vi "SwapInstanceVIUnusedName2 61.vi"(6 "Bindata & descr in":T1, 7 "type":i16, 8 "error in (no error)":errorcluster, 9 "dims":u8=3 min=1 max=3, 11 "kwarg_name":string="testarg") -> (0 "error out":errorcluster, 1 "Array 3D":i16[][][](array[numeric]), 2 "Array 2D":i16[][](array[numeric]), 3 "Array 1D":i16[](array[numeric]), 4 "Bindata & descr out":T1, 5 "bindata":u8[](array[numeric]))   [LabVIEW 2018]
uses:
  Bindata&description.ctl
  Bindata description.ctl
  7506c77e-6b82-4e17-9890-cbd22e6c05b4.vi
  f7386c90-d632-48db-ac3f-67c7d297baaf.vi
  c9ce9a8f-9ac7-4987-9358-ae921b7c55ea.vi
  f51c2130-6ae0-4021-866b-c8a633ea51c1.vi
  f7386c90-d632-48db-ac3f-67c7d297baaf.vi/c5b35af8-591a-407a-bd5b-5a277ce86d41.vi
  c9ce9a8f-9ac7-4987-9358-ae921b7c55ea.vi/6c170469-4803-4e09-bad0-e8de8ae58185.vi
  f51c2130-6ae0-4021-866b-c8a633ea51c1.vi/17c796ad-9fc0-4ce8-a0f5-ba301a22375f.vi
  f7386c90-d632-48db-ac3f-67c7d297baaf.vi/c5b35af8-591a-407a-bd5b-5a277ce86d41.vi/1233fed4-38f0-45f0-9b08-281c3922a2b5.vi
  c9ce9a8f-9ac7-4987-9358-ae921b7c55ea.vi/6c170469-4803-4e09-bad0-e8de8ae58185.vi/b23d98bf-518b-4b7c-8067-e1a442489f46.vi
  f51c2130-6ae0-4021-866b-c8a633ea51c1.vi/17c796ad-9fc0-4ce8-a0f5-ba301a22375f.vi/a95c6ce7-26be-4e62-abca-42e88a52b093.vi
  f7386c90-d632-48db-ac3f-67c7d297baaf.vi/c5b35af8-591a-407a-bd5b-5a277ce86d41.vi/1233fed4-38f0-45f0-9b08-281c3922a2b5.vi/90a762d1-1a34-427c-b834-b42d639573de.vi
  c9ce9a8f-9ac7-4987-9358-ae921b7c55ea.vi/6c170469-4803-4e09-bad0-e8de8ae58185.vi/b23d98bf-518b-4b7c-8067-e1a442489f46.vi/8554908a-2c98-41e5-8847-754fe8ddb4a9.vi
  f51c2130-6ae0-4021-866b-c8a633ea51c1.vi/17c796ad-9fc0-4ce8-a0f5-ba301a22375f.vi/a95c6ce7-26be-4e62-abca-42e88a52b093.vi/24253328-9668-44c3-b88c-e275f2342f8c.vi
  check ID validity.vi
  LV-Julia_ZMQ-Roundtrip_lib.lvlib
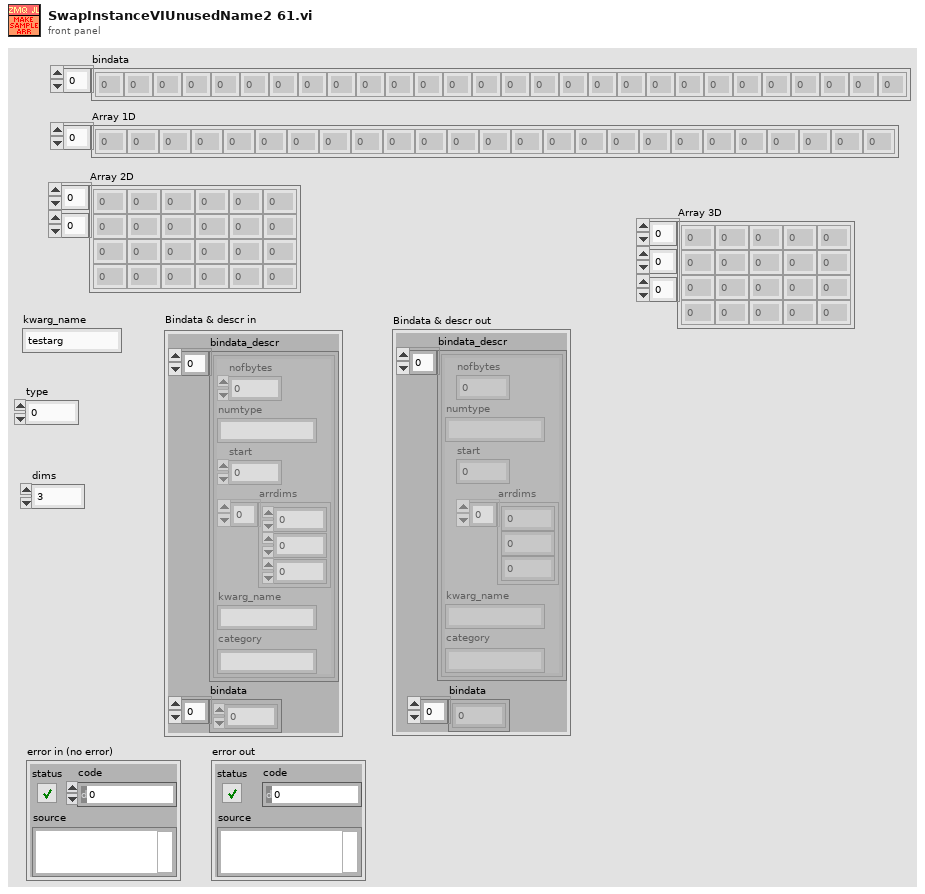
[diagram p1: front panel]
types:
  T1 = typedef "Bindata&description.ctl" = cluster{"bindata_descr":T2[], "bindata":u8[]}
  T2 = typedef "LV-Julia_ZMQ-Roundtrip_lib.lvlib/Bindata description.ctl" = cluster{"nofbytes":i32, "numtype":string, "start":i32, "arrdims":i32[], "kwarg_name":string, "category":string}
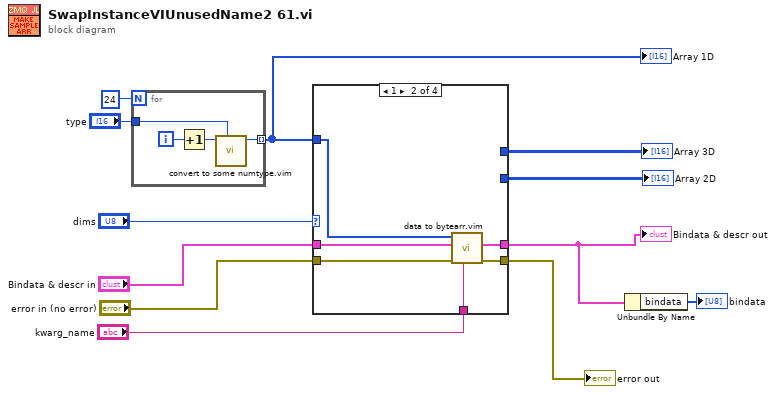
[diagram p0: block diagram]
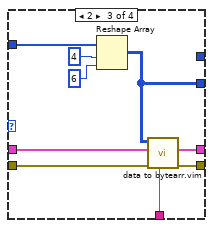
[diagram p3: hidden frame]
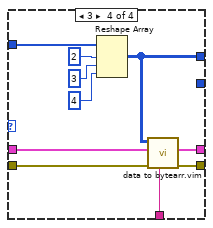
[diagram p4: hidden frame]
diagram:
  n1 = for {
    N: 24 -> [_]
    tunnel: [w14] -> w11 mode=indexing
    tunnel: "type" -> [w13]
    i -> [w16]
    n2 = Increment(x=w16) -> (x+1=w15:i32)
    n3 = call "convert to some numtype.vim"("type"=w13, "Numeric in"=w15) -> ("Numeric out"=w14:i16)  [unwired: 9 in]
  }
  "Array 1D" <- w11
  n4 = case shown="1" "dims" {
    tunnel: [_ _ _ w42] -> w12
    tunnel: w11 -> [_ w23 w30 w38]
    tunnel: "kwarg_name" -> [_ w22 w29 w37]
    tunnel: "error in (no error)" -> [w17 w21 w28 w36]
    tunnel: [w17 w20 w27 w35] -> w5
    tunnel: [_ w19 w26 w34] -> w2
    tunnel: [_ _ w25 _] -> w4
    tunnel: "Bindata & descr in" -> [_ w18 w24 w33]
    frame 0, Default {
    }
    frame 1 {
      n5 = call "data to bytearr.vim"("kwarg_name"=w22, "error in (no error)"=w21, "Bindata & descr in"=w18, "data in"=w23) -> ("error out"=w20:errorcluster, "Bindata & descr out"=w19:T1)  [unwired: 5 in, 1 out]
    }
    frame 2 {
      n6 = Reshape Array(w30, 4 ("dimension size"), 6 ("dimension size")) -> (w25:i16[][])
      n7 = call "data to bytearr.vim"("kwarg_name"=w29, "error in (no error)"=w28, "Bindata & descr in"=w24, "data in"=w25) -> ("error out"=w27:errorcluster, "Bindata & descr out"=w26:T1)  [unwired: 5 in, 1 out]
    }
    frame 3 {
      n8 = Reshape Array(w38, 2 ("dimension size"), 3 ("dimension size"), 4 ("dimension size")) -> (w42:i16[][][])
      n9 = call "data to bytearr.vim"("kwarg_name"=w37, "error in (no error)"=w36, "Bindata & descr in"=w33, "data in"=w42) -> ("error out"=w35:errorcluster, "Bindata & descr out"=w34:T1)  [unwired: 5 in, 1 out]
    }
  }
  "Array 3D" <- w12
  "Bindata & descr out" <- w2
  "error out" <- w5
  "Array 2D" <- w4
  n10 = Unbundle By Name(w2) -> ("bindata"=→"bindata":u8[])
